vi "BuyProduct.vi"(8 "error in (no error)":errorcluster, 10 "Comprar":bool, 11 "Coca Actors in":refnum<class "Coca Actors.lvclass">) -> (0 "error out":errorcluster, 3 "Coca Actors out":refnum<class "Coca Actors.lvclass">)   [LabVIEW 2020, in "Coca Actors.lvlib" / "Coca Actors.lvclass"]
uses:
  Coca Actors.lvclass
  Coca Actors.lvclass/Coca Actors.ctl
panel:
  out "output cluster":T1
  in  "Cluster":T1
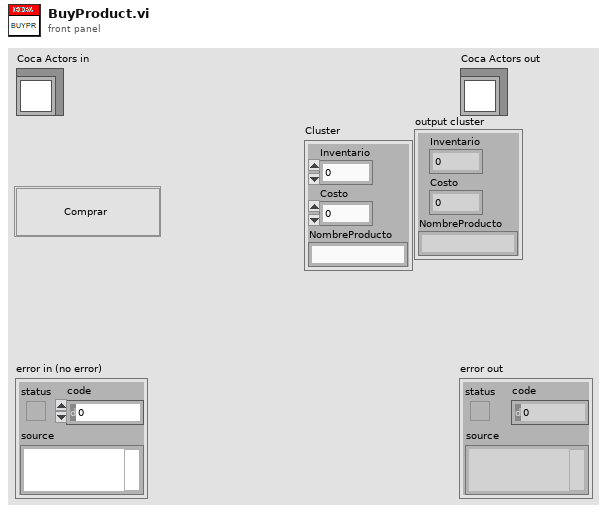
[diagram p1: front panel]
types:
  T1 = cluster{"Inventario":i32, "Costo":dbl, "NombreProducto":string}
  T2 = cluster{"Data[0]":string, "Data[1]":string, "Data[2]":string, "Data[3]":string, "Data[4]":string, "Data[5]":string, "Data[6]":string, "Data[7]":string, "Data[8]":string}
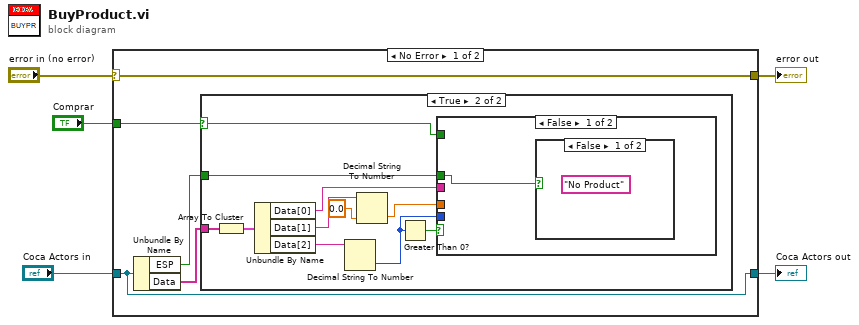
[diagram p0: block diagram]
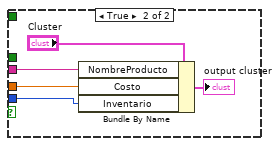
[diagram p4: hidden frame]
diagram:
  n1 = case shown="No Error" "error in (no error)" {
    selector: "error in (no error)" -> [w10 w29]
    tunnel: [w10 w29] -> w4
    tunnel: [w9 w28] -> w2
    tunnel: "Coca Actors in" -> [w9 w28]
    tunnel: "Comprar" -> [w8 _]
    frame No Error {
      n2 = Unbundle By Name(w9) -> ("ESP"=w6:bool, "Data"=w7:string[])
      n3 = case shown="True" w8 {
        selector: w8 -> [_ w11]
        tunnel: w7 -> [_ w21]
        tunnel: w6 -> [_ w16]
        frame False {
        }
        frame True {
          n4 = Array To Cluster(array=w21) -> (cluster=w20:T2)
          n5 = Unbundle By Name(w20) -> ("Data[0]"=w13:string, "Data[1]"=w19:string, "Data[2]"=w17:string)
          n6 = Decimal String To Number(string=w17) -> (number=w12:i32)  [unwired: 2 in, 1 out]
          n7 = Decimal String To Number(string=w19, default (0L)=0.0) -> (number=w14:dbl)  [unwired: 1 in, 1 out]
          n8 = Greater Than 0?(x=w12) -> (x > 0?=w15:bool)
          n9 = case shown="False" w15 {
            tunnel: w14 -> [_ w25]
            tunnel: w16 -> [w22 _]
            tunnel: w13 -> [_ w26]
            tunnel: w12 -> [_ w24]
            tunnel: w11 -> [_ _]
            frame False {
              n10 = case shown="False" w22 {
                frame False {
                  (unwired) "No Product"
                }
                frame True {
                }
              }
            }
            frame True {
              n11 = Bundle By Name(cluster="Cluster", "NombreProducto"=w26, "Costo"=w25, "Inventario"=w24) -> (→"output cluster":T1)
            }
          }
        }
      }
    }
    frame Error {
    }
  }
  "error out" <- w4
  "Coca Actors out" <- w2
